vi "Memory.Pointer.Write.0D.U64.No Check.vi"(8 "error in (no error)":errorcluster, 9 "offset (0)":u64 format="%d bytes", 10 "value":u64, 11 "pointer in":refnum<class "Memory.Pointer.lvclass">) -> (0 "error out":errorcluster, 1 "offset out":u64 format="%d bytes", 2 "value":u64, 3 "pointer out":refnum<class "Memory.Pointer.lvclass">)   [LabVIEW 2016, in "Memory.lvlib" / "Memory.Pointer.lvclass"]
doc: "Writes the provided <b>value</b> to the address specified by <b>pointer + offset</b>.\n\n<b>Note:</b> This VI is <b>unsafe</b>.\n\nUnsafe means that it does not evaluate the size parameter of <b>pointer</b> to ensure that is inbounds of allocated memory before peforming a memory read/write. Reading/writing more data to a pointer than it has allocated can corrupt or crash LabVIEW. Only use this VI in scenarios where the <b>pointer</b> has been validated to be allocated to a correct size before calling this VI."
uses:
  Memory.Pointer.lvclass
  Memory.Pointer.lvclass/Memory.Pointer.ctl
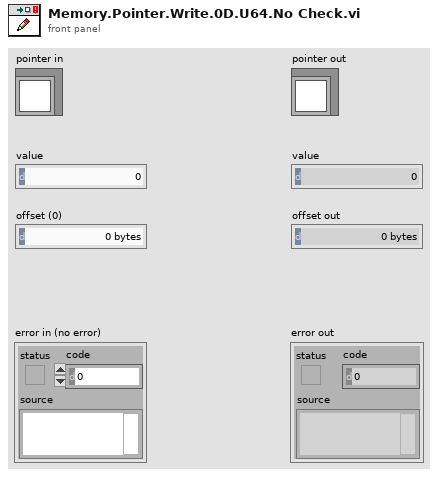
[diagram p1: front panel]
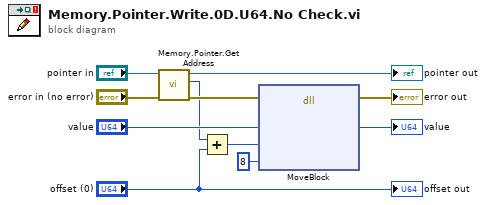
[diagram p0: block diagram]
diagram:
  n1 = call "Memory.Pointer.Get Address.vi"("Pointer in"="pointer in") -> ("address"=w1:u64, "Pointer out"=→"pointer out":refnum<class "Memory.Pointer.lvclass">)  [unwired: 9 in]
  n2 = Add(x=w1, y="offset (0)") -> (x+y=w4:u64)
  n3 = dll-call lib="LabVIEW" fn="MoveBlock"(error in="error in (no error)", "src"="value", "dst"=w4, "size"=u64 8) -> (error out=→"error out":errorcluster, "src"=→"value":u64)  [unwired: 5 in, 1 out]
  "offset out" <- "offset (0)"
